vi "UsrProfiles-Source-Default user button text.vi"() -> (1 "Default user boolean text constant":string)   [LabVIEW 2020]
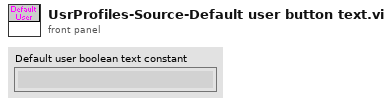
[diagram p1: front panel]
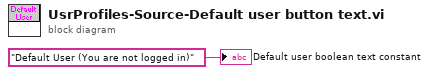
[diagram p0: block diagram]
diagram:
  "Default user boolean text constant" <- "Default User (You are not logged in)"
